vi "picture_to_frame_array.vi"(1 "Image In":cluster{"X":dbl, "Y":dbl}[][](array[cluster])) -> (0 "Image Out":cluster{"X":dbl, "Y":dbl, "Laser":bool}[](array[cluster]))   [LabVIEW 2017]
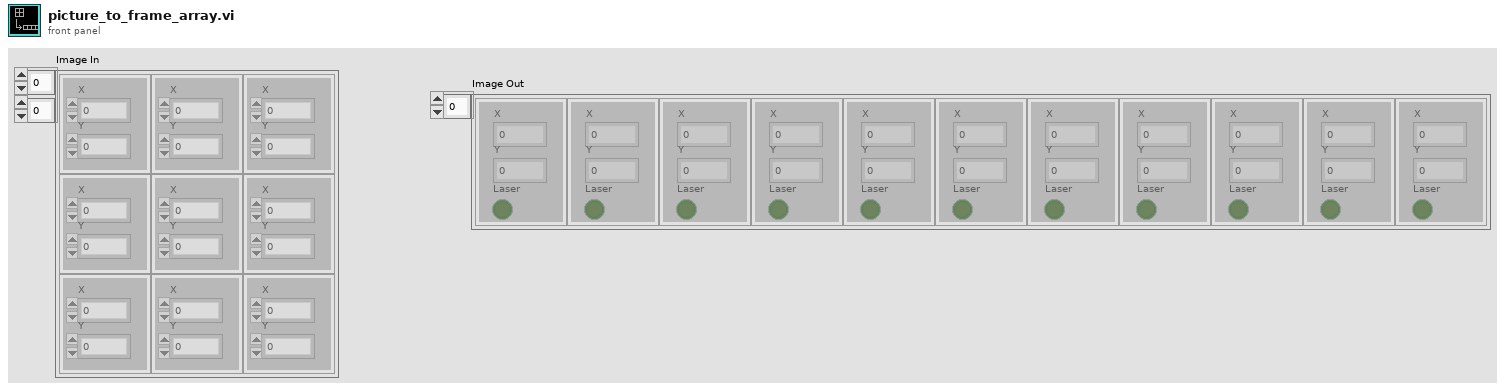
[diagram p1: front panel]
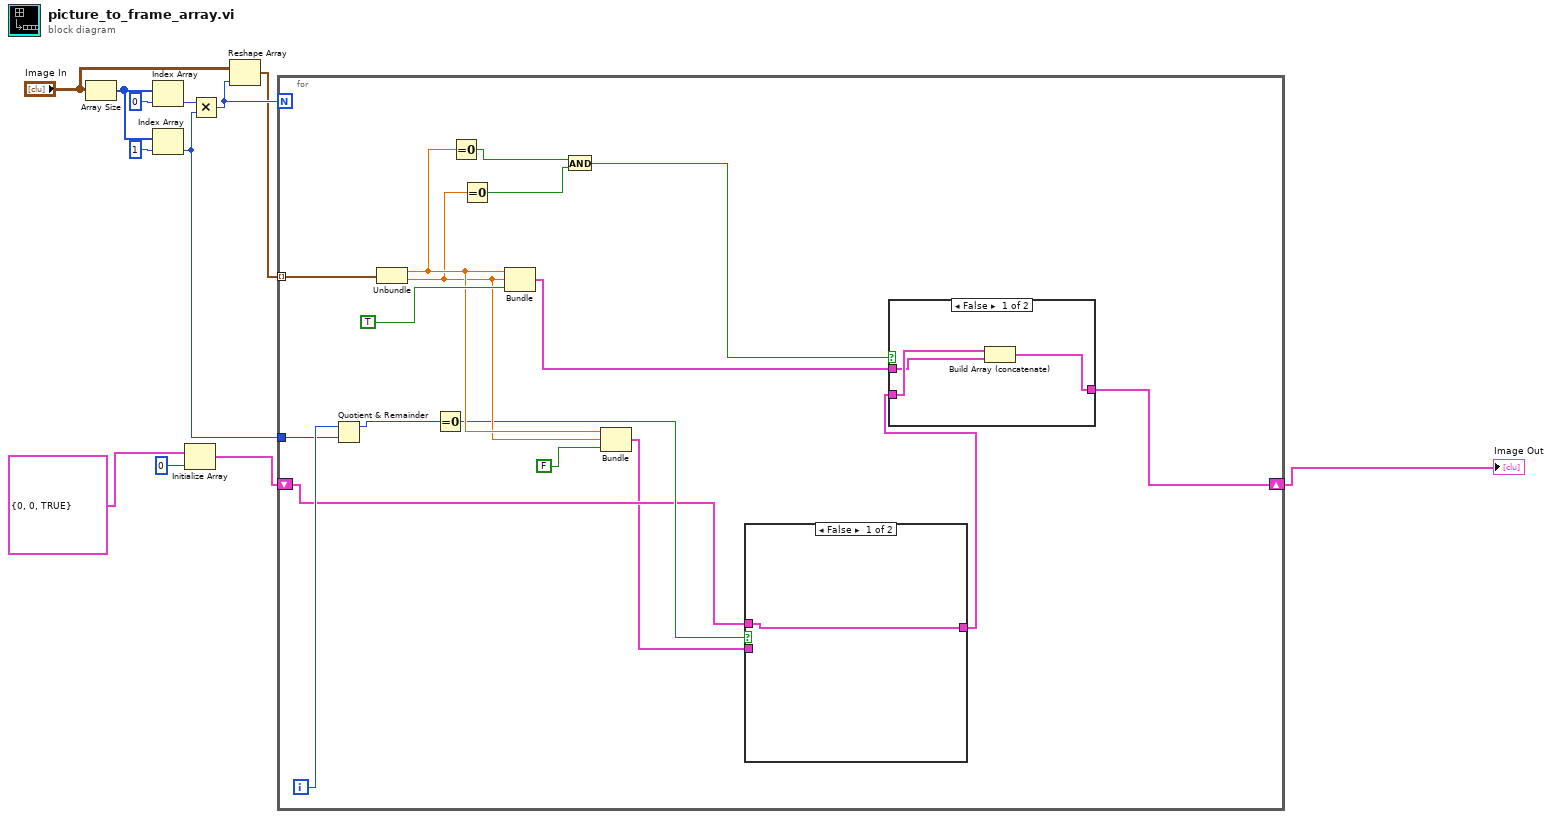
[diagram p0: block diagram]
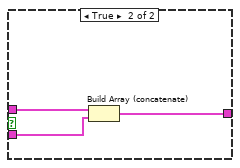
[diagram p2: hidden frame]
diagram:
  n1 = Array Size(array="Image In") -> (size(s)=w12:i32[])
  n2 = Index Array(array=w12, index=0) -> (element=w2:i32)
  n3 = Index Array(array=w12, index=1) -> (element=w1:i32)
  n4 = Initialize Array(cluster{i32, i32, bool} {0, 0, TRUE}, 0 ("dimension size")) -> (w4:cluster{i32, i32, bool}[])
  n5 = Multiply(x=w2, y=w1) -> (x*y=w8:i32)
  n6 = Reshape Array("Image In", w8) -> (w7:cluster{"X":dbl, "Y":dbl}[])
  n7 = for {
    N: w8 -> [_]
    shift-right: [w17] -> w3
    shift-left: w4 -> [w16]
    tunnel: w7 -> [w29] mode=indexing
    tunnel: w1 -> [w13]
    i -> [w24]
    n8 = Quotient & Remainder(x=w24, y=w13) -> (x-y*floor(x/y)=w23:i32)  [unwired: 1 out]
    n9 = Unbundle(w29) -> ("X"=w20:dbl, "Y"=w19:dbl)
    n10 = Equal To 0?(x=w23) -> (x = 0?=w18:bool)
    n11 = Equal To 0?(x=w20) -> (x = 0?=w27:bool)
    n12 = Equal To 0?(x=w19) -> (x = 0?=w26:bool)
    n13 = Bundle("X"=w20, "Y"=w19, TRUE) -> (w22:cluster{"X":dbl, "Y":dbl, bool})  [unwired: 1 in]
    n14 = And(x=w27, y=w26) -> (x .and. y?=w25:bool)
    n15 = Bundle("X"=w20, "Y"=w19, FALSE) -> (w15:cluster{"X":dbl, "Y":dbl, bool})  [unwired: 1 in]
    n16 = case shown="False" w18 {
      tunnel: w16 -> [w30 w33]
      tunnel: w15 -> [_ w32]
      tunnel: [w30 w31] -> w14
      frame False {
      }
      frame True {
        n17 = Build Array (concatenate)(w33, w32) -> (w31:cluster{"X":dbl, "Y":dbl, bool}[])
      }
    }
    n18 = case shown="False" w25 {
      tunnel: [w34 w37] -> w17
      tunnel: w14 -> [w36 w37]
      tunnel: w22 -> [w35 _]
      frame False {
        n19 = Build Array (concatenate)(w36, w35) -> (w34:cluster{"X":dbl, "Y":dbl, bool}[])
      }
      frame True {
      }
    }
  }
  "Image Out" <- w3
